vi "Real-Time Main.vi"() -> ()   [LabVIEW 2024]
uses:
  <vilib>/platform/TimedLoop/XDataNode/XDataNode.xnode
  <vilib>/Platform/TimedLoop/XDataNode/nitl_modes.ctl
  <vilib>/Platform/TimedLoop/XDataNode/XDNodeRunTimeDep.lvlib
  <vilib>/Platform/TimedLoop/XDataNode/wakeup.ctl
  <vilib>/Platform/TimedLoop/XDataNode/timing_clust.ctl
panel:
  out "error out":errorcluster
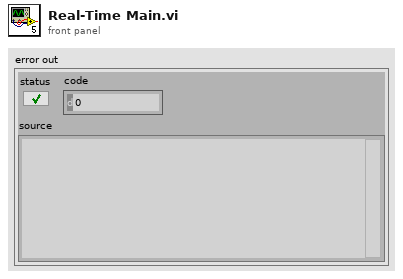
[diagram p1: front panel]
types:
  T1 = typedef "XDNodeRunTimeDep.lvlib/timing_clust.ctl" = cluster{"Expected End [f-1]":u64, "Actual End [f-1]":u64, "Finished Late? [f-1]":bool, "Expected End [i-1]":u64, "Actual End [i-1]":u64, "Finished Late? [i-1]":bool, "Expected Start [i]":u64, "Actual Start [i]":u64, "Expected Start [f]":u64, "Actual Start [f]":u64, "Source Name":string, "Structure Name":string, "Period":i64, "Deadline":i64, "Offset":i64, "Start":i64, "Priority":i32, "Timeout":i32, "Mode":T2, "Wakeup Reason":T3, "Error":errorcluster, "Source Type":string, "Secondary Source Type":string, "Global End Time":u64, "Global Start Time":u64, "Frame Duration":u64, "Iteration Duration":u64, "Assigned CPU":i32, "I/O Scan Engine Mode":u32}
  T2 = typedef "XDNodeRunTimeDep.lvlib/nitl_modes.ctl" = enum32{"No Change", "Process missed periods, maintain original phase", "Discard missed periods, maintain original phase", "Process missed periods, ignore original phase", "Discard missed periods, ignore original phase"}
  T3 = typedef "XDNodeRunTimeDep.lvlib/wakeup.ctl" = enum32{"Normal", "Aborted", "Asynchronous wakeup", "Timing source error", "Timed loop error", "Timeout"}
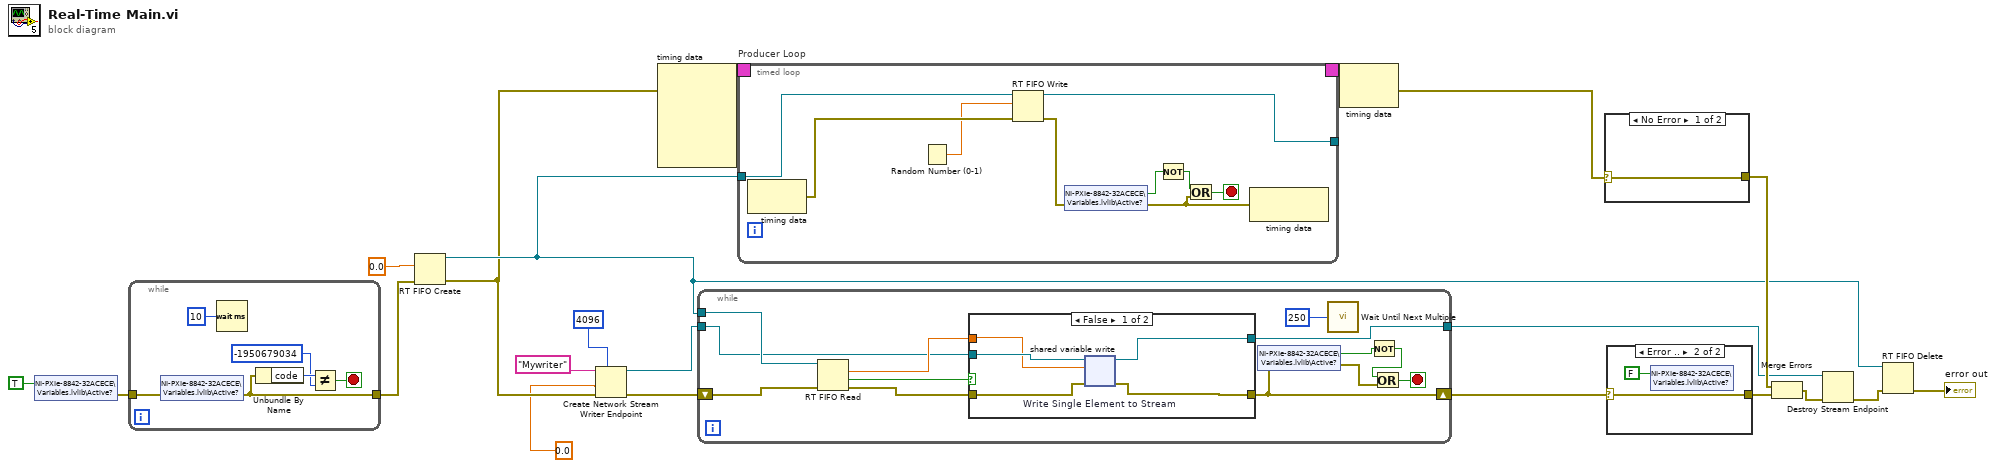
[diagram p0: block diagram]
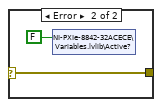
[diagram p3: hidden frame]
diagram:
  n1 = shared-variable "NI-PXIe-8842-32ACECE\\Variables.lvlib\\Active?"(TRUE) -> (error out=w17:errorcluster)  [unwired: 1 in]
  n2 = while {
    tunnel: w17 -> [w27]
    tunnel: [w22] -> w16
    stop <- w24 stop-if-true
    n3 = shared-variable "NI-PXIe-8842-32ACECE\\Variables.lvlib\\Active?"(error in=w27) -> (error out=w22:errorcluster)  [unwired: 1 out]
    n4 = Wait (ms)(milliseconds to wait=u32 10) -> ()  [unwired: 1 out]
    n5 = Unbundle By Name(w22) -> ("code"=w26:i32)
    n6 = Not Equal?(x=w26, y=-1950679034) -> (x != y?=w24:bool)
  }
  n7 = RT FIFO Create(1:0.0 ("datapoints in waveform (1)"), 3:w16) -> (8:w11:refnum<k33>, 11:w9:errorcluster)  [unwired: 6 in, 1 out]
  n8 = Create Network Stream Writer Endpoint(7:4096 ("writer buffer size"), 8:w9, 9:0.0, 11:"Mywriter" ("writer name")) -> (0:w10:errorcluster, 3:w7:refnum<k21>)  [unwired: 3 in]
  n9 = node-c288(w9) -> (w21:T1)  [unwired: 4 in]
  n10 = while {
    tunnel: w11 -> [w31]
    shift-right: [w32] -> w13
    shift-left: w10 -> [w37]
    tunnel: w7 -> [w29]
    tunnel: [w28] -> w3
    stop <- w33 stop-if-true
    n11 = RT FIFO Read(0:w31, 3:w37) -> (9:w39:dbl, 10:w40:bool, 11:w38:errorcluster)  [unwired: 2 in, 2 out]
    n12 = case shown="False" w40 {
      tunnel: w39 -> [w42 _]
      tunnel: [w44 w47] -> w32
      tunnel: w38 -> [w45 w47]
      tunnel: w29 -> [w43 w46]
      tunnel: [w41 w46] -> w28
      frame False {
        n13 = shared-variable-write "Write Single Element to Stream"(w43, w45, w42) -> (w41:refnum<k21>, w44:errorcluster)  [unwired: 1 in, 1 out]
      }
      frame True {
      }
    }
    n14 = shared-variable "NI-PXIe-8842-32ACECE\\Variables.lvlib\\Active?"(error in=w32) -> (w36:bool, error out=w34:errorcluster)
    n15 = call "Wait Until Next Multiple"("Count(mSec)"=u32 250) -> ()  [unwired: 1 out]
    n16 = Not(x=w36) -> (.not. x?=w35:bool)
    n17 = Or(x=w35, y=w34) -> (x .or. y?=w33:bool)
  }
  n18 = timed-loop "Producer Loop" {
    timing: w21 -> [_]
    timing-out: [_] -> w20
    tunnel: w11 -> [w49]
    tunnel: [w48] -> _
    stop <- w51 stop-if-true
    n19 = node-c288() -> (w56:errorcluster)  [unwired: 1 in]
    n20 = Random Number (0-1)() -> (number: 0 to 1=w55:dbl)
    n21 = RT FIFO Write(0:w49, 1:w55, 3:w56) -> (8:w48:refnum<k33>, 11:w54:errorcluster)  [unwired: 2 in, 2 out]
    n22 = shared-variable "NI-PXIe-8842-32ACECE\\Variables.lvlib\\Active?"(error in=w54) -> (w53:bool, error out=w50:errorcluster)
    n23 = Not(x=w53) -> (.not. x?=w52:bool)
    n24 = Or(x=w52, y=w50) -> (x .or. y?=w51:bool)
    n25 = node-c288(w50) -> ()  [unwired: 1 out]
  }
  n26 = node-c288(w20) -> (w15:errorcluster)
  n27 = case shown="No Error" w15 {
    selector: w15 -> [w62 w63]
    tunnel: [w62 w63] -> w14
    frame No Error {
    }
    frame Error {
      n28 = shared-variable "NI-PXIe-8842-32ACECE\\Variables.lvlib\\Active?"(FALSE) -> ()  [unwired: 1 in, 1 out]
    }
  }
  n29 = case shown="Error .." w13 {
    selector: w13 -> [w65 w66]
    tunnel: [w65 w66] -> w12
    frame No Error {
    }
    frame Error {
      n30 = shared-variable "NI-PXIe-8842-32ACECE\\Variables.lvlib\\Active?"(FALSE) -> ()  [unwired: 1 in, 1 out]
    }
  }
  n31 = Merge Errors(w14, w12) -> (w5:errorcluster)
  n32 = Destroy Stream Endpoint(8:w5, 11:w3) -> (0:w6:errorcluster)
  n33 = RT FIFO Delete(0:w11, 3:w6) -> (11:→"error out":errorcluster)  [unwired: 1 in]
